vi "Sample_positions_to_table.vi"(1 "Sample Positions array":T1[](array[typedef]) {"Z" format="%.1f"; "Y" format="%.1f"; "X" format="%.1f"; "SAMPLE NO." min=1 max=40 step=1}) -> (0 "Table":string[][](table))   [LabVIEW 2010]
uses:
  Controls/Sample_pos.ctl
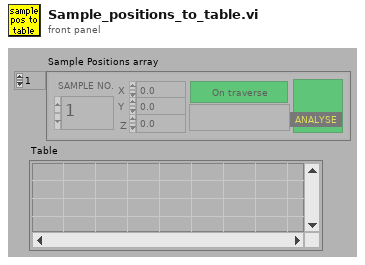
[diagram p1: front panel]
types:
  T1 = typedef "Sample_pos.ctl" = cluster{"SAMPLE NO.":i32, "X":dbl, "Y":dbl, "Z":dbl, "On trav":bool, "Analyse?":bool, "Notes":string}
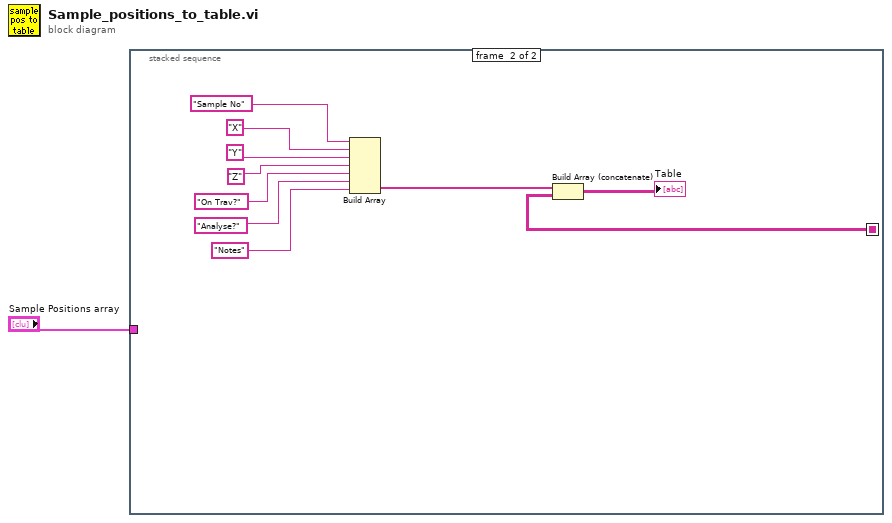
[diagram p0: block diagram]
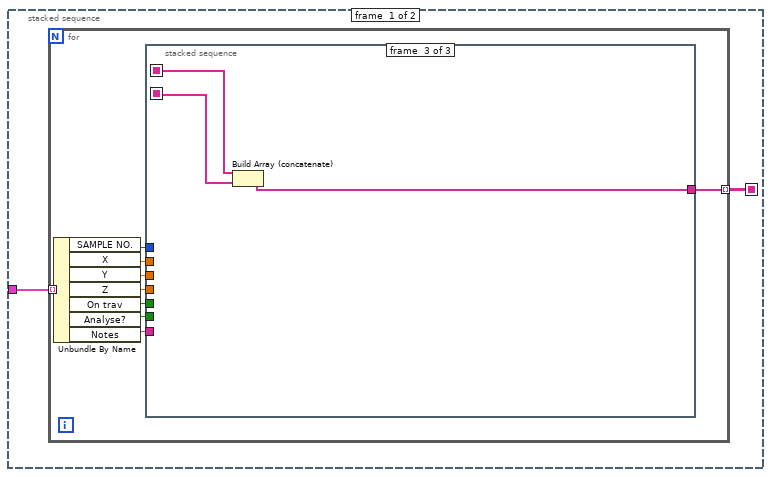
[diagram p2: hidden frame]
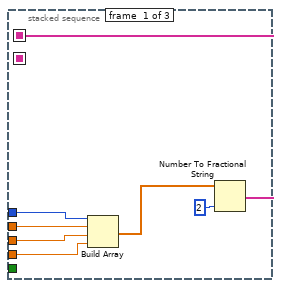
[diagram p3: hidden frame]
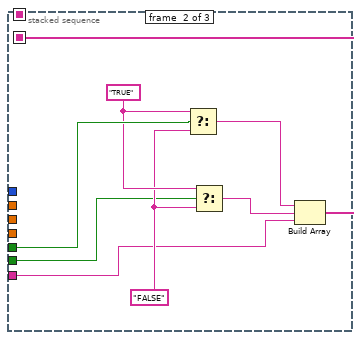
[diagram p4: hidden frame]
diagram:
  n1 = stacked-sequence {
    seq-local: [w2 _] -> [_ w32]
    tunnel: "Sample Positions array" -> [w3 _]
    frame #0 {
      n2 = for {
        tunnel: w3 -> [w12] mode=indexing
        tunnel: [w4] -> w2 mode=indexing
        n3 = Unbundle By Name(w12) -> ("SAMPLE NO."=w11:i32, "X"=w10:dbl, "Y"=w9:dbl, "Z"=w8:dbl, "On trav"=w7:bool, "Analyse?"=w6:bool, "Notes"=w5:string)
        n4 = stacked-sequence {
          seq-local: [w18 _ _] -> [_ _ w30]
          seq-local: [_ w26 _] -> [_ _ w29]
          tunnel: w11 -> [w17 _ _]
          tunnel: w10 -> [w16 _ _]
          tunnel: w9 -> [w15 _ _]
          tunnel: w8 -> [w14 _ _]
          tunnel: w7 -> [_ w25 _]
          tunnel: w6 -> [_ w22 _]
          tunnel: w5 -> [_ w20 _]
          tunnel: [_ _ w28] -> w4
          frame #0 {
            n5 = Build Array(w17, w16, w15, w14) -> (w13:dbl[])
            n6 = Number To Fractional String(number=w13, precision (6)=i16 2) -> (F-format string=w18:string[])  [unwired: 2 in]
          }
          frame #1 {
            w23 = "FALSE"
            w24 = "TRUE"
            n7 = Select(t=w24, s=w25, f=w23) -> (s? t:f=w27:string)
            n8 = Select(t=w24, s=w22, f=w23) -> (s? t:f=w21:string)
            n9 = Build Array(w27, w21, w20) -> (w26:string[])
          }
          frame #2 {
            n10 = Build Array (concatenate)(w30, w29) -> (w28:string[])
          }
        }
      }
    }
    frame #1 {
      n11 = Build Array("Sample No", "X", "Y", "Z", "On Trav?", "Analyse?", "Notes") -> (w33:string[])
      n12 = Build Array (concatenate)(w33, w32) -> (→"Table":string[][])
    }
  }
